vi "Motor_PNWrite_CableTensionRef.vi"(8 "error in (no error)":errorcluster, 10 "CableTensionRef":dbl[](array[numeric]), 11 "MotorControl in":refnum<class "MotorControl.lvclass">) -> (0 "error out":errorcluster, 3 "MotorControl out":refnum<class "MotorControl.lvclass">)   [LabVIEW 2015, in "MotorControl.lvclass"]
uses:
  MotorControl.lvclass
  MotorControl.lvclass/MotorControl.ctl
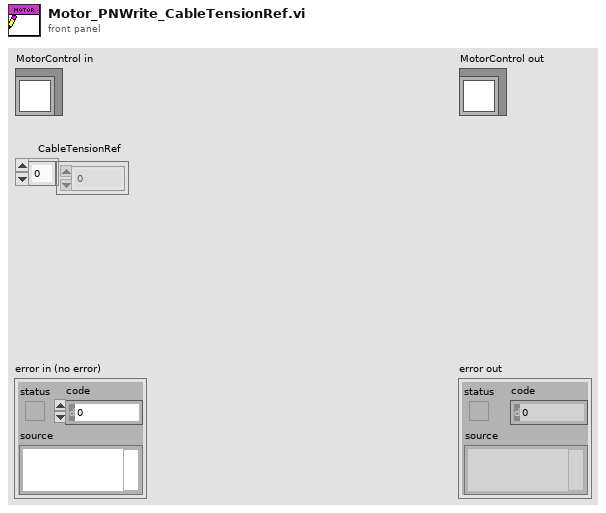
[diagram p1: front panel]
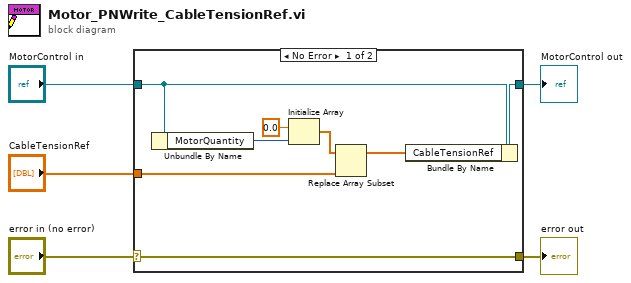
[diagram p0: block diagram]
diagram:
  n1 = case shown="No Error" "error in (no error)" {
    selector: "error in (no error)" -> [w13 w14]
    tunnel: [w13 w14] -> w4
    tunnel: [w12 w15] -> w2
    tunnel: "MotorControl in" -> [w11 w15]
    tunnel: "CableTensionRef" -> [w7 _]
    frame No Error {
      n2 = Unbundle By Name(w11) -> ("MotorQuantity"=w10:i32)
      n3 = Initialize Array(0.0 ("element"), w10) -> (w8:dbl[])
      n4 = Replace Array Subset(array=w8, new element=w7) -> (w6:dbl[])  [unwired: 1 in]
      n5 = Bundle By Name(cluster=w11, "CableTensionRef"=w6) -> (w12:refnum<class "MotorControl.lvclass">)
    }
    frame Error {
    }
  }
  "error out" <- w4
  "MotorControl out" <- w2
